vi "Save_WeldAuto_Recipe.vi"(6 "Message ID":dbl, 8 "Error IN":errorcluster, 9 "Parameter Key values":i16[](array[numeric]), 10 "Response ID":u8=66, 11 "connection ID":refnum<k5>) -> (1 "Error OUT":errorcluster, 2 "Test status":string=" Success", 3 "connection ID":refnum<k5>)   [LabVIEW 2017]
panel:
  out "String value response":string
  out "*(type *) &x 2":u8
  out "*(type *) &x":u8
  out "bytes written":i32
  # "INPUT"
  # "OUTPUT"
  # "Read Me:\nThis VI will send the set of recipe parameters to \nSC BL and verifies the response recieved from the SCBL"
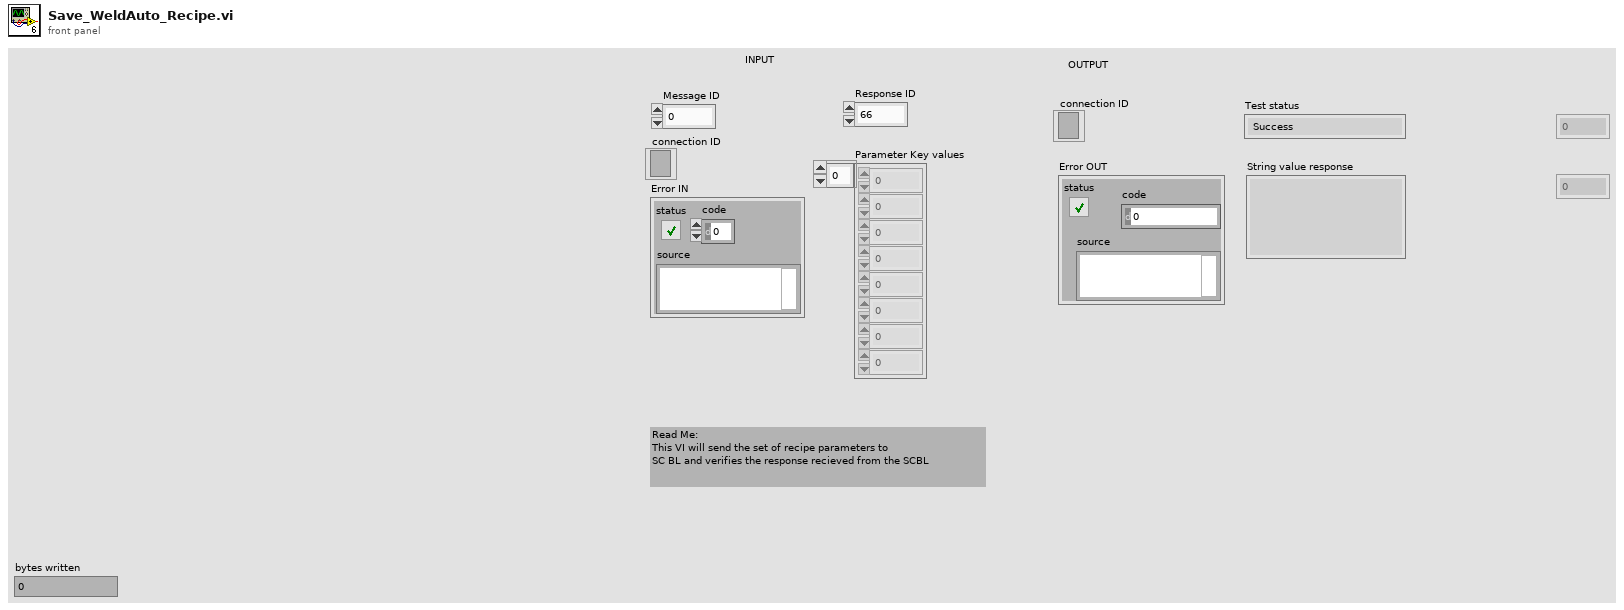
[diagram p1: front panel]
types:
  T1 = enum16{"big-endian, network order", "native, host order", "little-endian"}
  T2 = cluster{"Parameter Key values":i16[], i32, "Message ID":dbl}
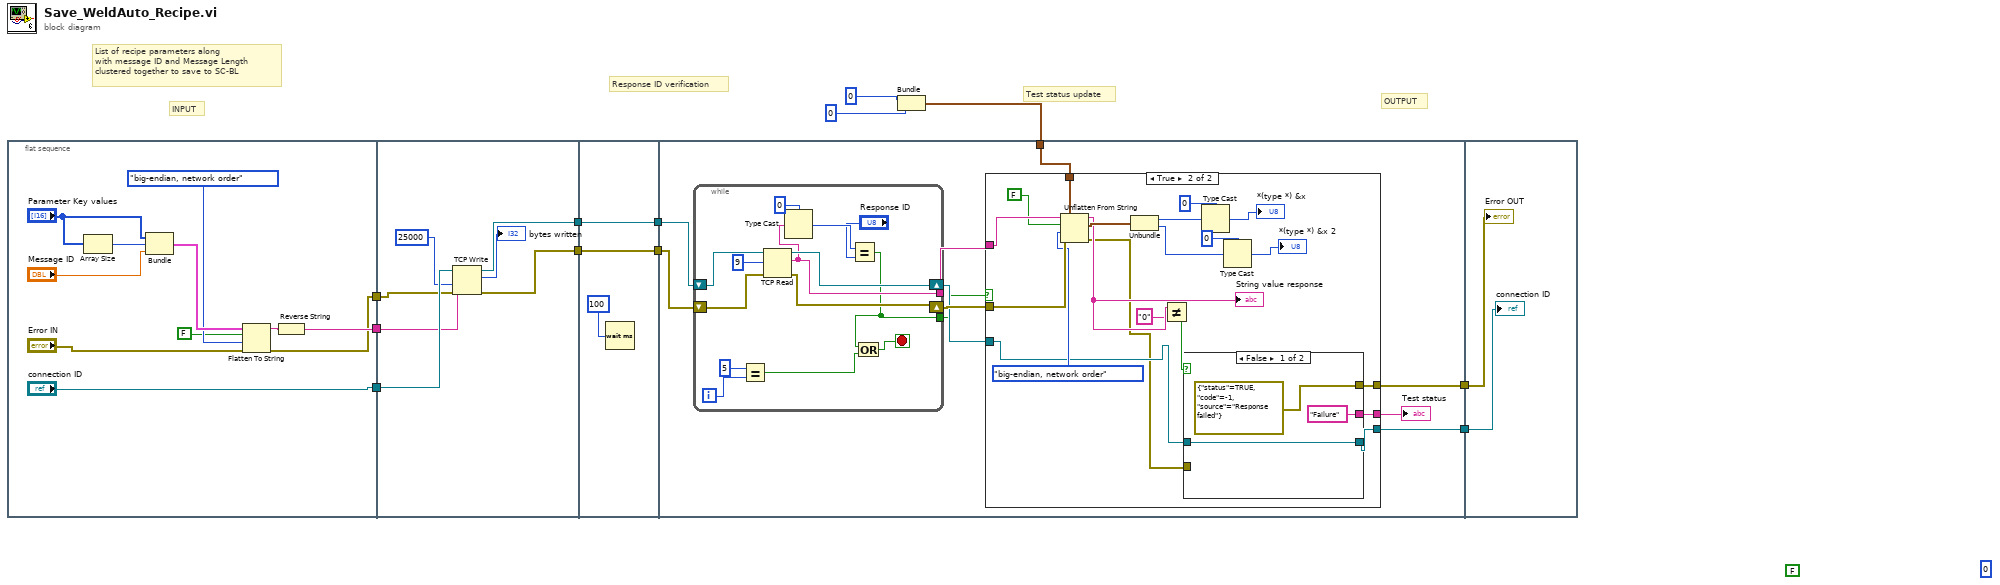
[diagram p0: block diagram]
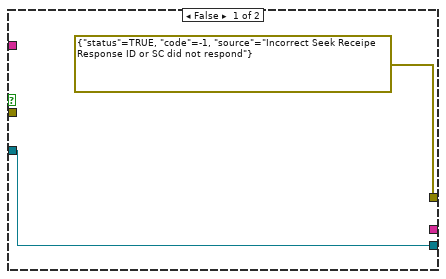
[diagram p2: hidden frame]
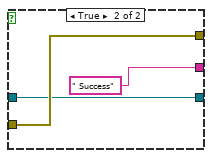
[diagram p3: hidden frame]
diagram:
  (unwired) u8 0
  (unwired) FALSE ("data includes array or string size? (T)")
  # "INPUT"
  # "List of recipe parameters along \nwith message ID and Message Length \nclustered together to save to SC-BL"
  # "OUTPUT"
  # "Test status update"
  # "Response ID verification"
  n1 = flat-sequence {
    tunnel: ["connection ID"] -> w3
    tunnel: [w13] -> w2
    tunnel: [w14] -> w1
    tunnel: [w30] -> w12
    tunnel: [w29] -> w11
    tunnel: w3 -> [w28]
    tunnel: w2 -> [w27]
    tunnel: w1 -> [w26]
    tunnel: w12 -> [w33]
    tunnel: w11 -> [w32]
    tunnel: [w33] -> w10
    tunnel: [w32] -> w9
    tunnel: w10 -> [w43]
    tunnel: w9 -> [w42]
    tunnel: w6 -> [w37]
    tunnel: [w36] -> w5
    tunnel: [w35] -> w4
    tunnel: w5 -> [w87]
    tunnel: w4 -> [w86]
    frame #0 {
      n2 = Array Size(array="Parameter Key values") -> (size(s)=w22:i32)
      n3 = Bundle("Parameter Key values"="Parameter Key values", w22, "Message ID"="Message ID") -> (w23:T2)  [unwired: 1 in]
      n4 = Flatten To String(anything=w23, prepend array or string size? (T)=FALSE, byte order (0:big-endian, network order)=T1."big-endian, network order", error in (no error)="Error IN") -> (data string=w18:string, error out=w13:errorcluster)  [unwired: 1 out]
      n5 = Reverse String(1:w18) -> (0:w14:string)
    }
    frame #1 {
      n6 = TCP Write(connection ID=w28, data in=w26, error in (no error)=w27, 9:25000 ("timeout ms (25000)")) -> (connection ID out=w30:refnum<k5>, bytes written=→"bytes written":i32, error out=w29:errorcluster)
    }
    frame #2 {
      n7 = Wait (ms)(milliseconds to wait=u32 100) -> ()  [unwired: 1 out]
    }
    frame #3 {
      n8 = while {
        tunnel: [w81] -> w40
        shift-right: [w83] -> w39
        shift-left: w43 -> [w85]
        shift-right: [w77] -> w41
        shift-left: w42 -> [w84]
        tunnel: [w75] -> w38
        i -> [w74]
        stop <- w76 stop-if-true
        n9 = Equal?(x=5, y=w74) -> (x = y?=w72:bool)
        n10 = TCP Read(connection ID=w85, bytes to read=9, error in (no error)=w84) -> (connection ID out=w83:refnum<k5>, data out=w81:string, error out=w77:errorcluster)  [unwired: 2 in]
        n11 = Type Cast(type=u8 0, x=w81) -> (*(type *) &x=w79:u8)
        n12 = Equal?(x=w79, y="Response ID") -> (x = y?=w75:bool)
        n13 = Or(x=w75, y=w72) -> (x .or. y?=w76:bool)
      }
      n14 = case shown="True" w38 {
        tunnel: w41 -> [_ w65]
        tunnel: w40 -> [_ w64]
        tunnel: w39 -> [w45 w56]
        tunnel: w37 -> [_ w60]
        tunnel: [w45 w55] -> w36
        tunnel: [errorcluster {"status"=TRUE, "code"=-1, "source"="Incorrect Seek Receipe Response ID or SC did not respond"} ("error constant") w54] -> w35
        tunnel: [_ w53] -> w34
        frame False {
        }
        frame True {
          n15 = Unflatten From String(type=w60, binary string=w64, data includes array or string size? (T)=FALSE, byte order (0:big-endian, network order)=T1."big-endian, network order", error in (no error)=w65) -> (rest of the binary string=w59:string, value=w61:cluster{i32, i32}, error out=w52:errorcluster)
          "String value response" <- w59
          n16 = Unbundle(w61) -> (w51:i32, w46:i32)
          n17 = Not Equal?(x=w59, y="0") -> (x != y?=w57:bool)
          n18 = case shown="False" w57 {
            tunnel: [errorcluster {"status"=TRUE, "code"=-1, "source"="Response failed"} ("error constant") w70] -> w54
            tunnel: w56 -> [w67 w69]
            tunnel: [w67 w69] -> w55
            tunnel: ["Failure" " Success"] -> w53
            tunnel: w52 -> [_ w70]
            frame False {
            }
            frame True {
            }
          }
          n19 = Type Cast(type=u8 0, x=w51) -> (*(type *) &x=→"*(type *) &x":u8)
          n20 = Type Cast(type=u8 0, x=w46) -> (*(type *) &x=→"*(type *) &x 2":u8)
        }
      }
      "Test status" <- w34
    }
    frame #4 {
      "connection ID" <- w87
      "Error OUT" <- w86
    }
  }
  n21 = Bundle(0, 0) -> (w6:cluster{i32, i32})  [unwired: 1 in]
